vi "Drive Controller.vi"(8 "error in":errorcluster) -> ()   [LabVIEW 2020]
doc: "This VI executes continuously carrying out the current operation and responding to updates or new operation requests. It will often contain the timing or control code that is difficult to place directly in TeleOp. This VI generally opens all sensors and motors and isolates the rest of the robot code from knowing implementation details of how the operations are carried out."
uses:
  <vilib>/Rock Robotics/WPI/Framework/Completion Status.ctl
  Drive Setpoints.ctl
  Drive Operations.ctl
  <vilib>/Rock Robotics/WPI/SafetyOutput/WPI_SafetyOutputConfigMenu.ctl
  <vilib>/Rock Robotics/WPI/Utilities/WPI_GetSetVariantRefNum.vi
  <vilib>/Rock Robotics/Network Tables/NT Write Number.vi
panel:
  in  "Interactive Values":T1
  in  "Buttons":cluster{"Execute Cmd":bool, "Abort Cmd":bool}
  out "Command Timing":cluster{"Start Time (ms)":u32, "Iterations":i32}
  out "Status":T3
  out "Setpoints":T4(graph)
  out "Current\nCmd":string
  # "Tip: The graph shows the motor setpoints. It may also be helpful to observe inputs and sensor values.\nYou may also want to display tuning or debugging controls."
  # "Interactive Command: You may fill in the settings for a command\nand schedule it with the Execute button. You can observe and abort\nany command while fine tuning the code for the controller."
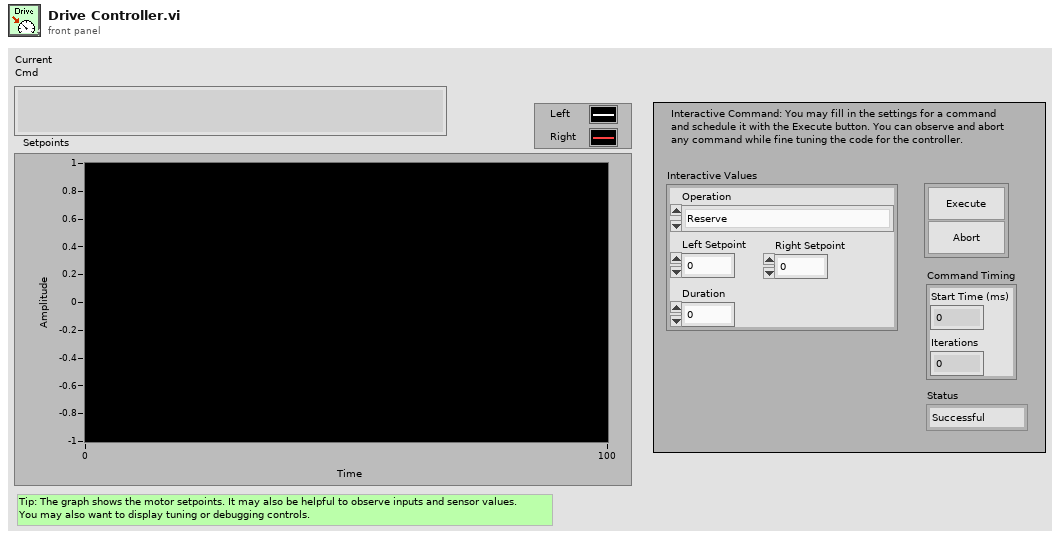
[diagram p1: front panel]
types:
  T1 = typedef "Drive Setpoints.ctl" = cluster{"Operation":T2, "Left Setpoint":dbl, "Right Setpoint":dbl, "Duration":dbl}
  T2 = typedef "Drive Operations.ctl" = enum16{"Reserve", "Read Current", "Immediate", "Drive for Time", "Drive for Distance"}
  T3 = typedef "Completion Status.ctl" = enum16{"Successful", "Aborted", "Incomplete"}
  T4 = cluster{"Left Setpoint":dbl, "Right Setpoint":dbl}
  T5 = typedef "WPI_SafetyOutputConfigMenu.ctl" = enum16{"Enable", "Disable"}
  T6 = typedef "WPI_RobotDriveDevRef.ctl" = cluster{"DevStatus":errorcluster, "Motors[]":T7[], "Square Inputs":bool, "Max Output":dbl}
  T7 = typedef "WPI_MotorControlDeviceRef.ctl" = cluster{"DeviceStatus":errorcluster, "Type":T8, "PWM":cluster{"PWM Channel":T9, "DeadBand":T10}, "CAN":cluster{"Device Number":u8, "SetOutput VI Ref":variant, "GetOutput VI Ref":variant, "Enable VI Ref":variant, "Disable VI Ref":variant, "Data":variant}, "Invert":bool, "DIO PWM":cluster{"PWM \"Enable\" Channel":T9, "DIOChannel":T11, "PWM Rate":dbl}}
  T8 = typedef "WPI_MotorControlType.ctl" = enum16{"PWM", "CAN", "DIO PWM"}
  T9 = typedef "FPGA_DIOPWMChannel.ctl" = enum8{"PWM 0", "PWM 1", "PWM 2", "PWM 3", "PWM 4", "PWM 5", "PWM 6", "PWM 7", "PWM 8", "PWM 9", "PWM MXP 0", "PWM MXP 1", "PWM MXP 2", "PWM MXP 3", "PWM MXP 4", "PWM MXP 5", "PWM MXP 6", "PWM MXP 7", "PWM MXP 8", "PWM MXP 9", "Invalid"}
  T10 = typedef "WPI_PWMDeadband.ctl" = cluster{"Name":string, "maxPositivePwm":i32, "minPositivePwm":i32, "centerPwm":i32, "maxNegativePwm":i32, "minNegativePwm":i32, "angularRange":u16}
  T11 = typedef "FPGA_DIOChannel.ctl" = enum8{"DIO 0", "DIO 1", "DIO 2", "DIO 3", "DIO 4", "DIO 5", "DIO 6", "DIO 7", "DIO 8", "DIO 9", "DIO MXP 0", "DIO MXP 1", "DIO MXP 2", "DIO MXP 3", "DIO MXP 4", "DIO MXP 5", "DIO MXP 6", "DIO MXP 7", "DIO MXP 8", "DIO MXP 9", "DIO MXP 10", "DIO MXP 11", "DIO MXP 12", "DIO MXP 13", "DIO MXP 14", "DIO MXP 15", "SPI Port CS1", "SPI Port CS2", "SPI Port CS3", "SPI Port MISO", "SPI Port MOSI", "Invalid"}
  T12 = typedef "Command Status Info.ctl" = cluster{"Name":string, "Status":T3, "notifier out":T13}
  T13 = typedef "Completion Notifier.ctl" = refnum<notifier>
  T14 = cluster{"SubSystem Data":T1, cluster{"Start Time (ms)":u32, "Iterations":i32}, cluster{"Command Info":T12, "Description":string, "Default Command":T1, "queue out":refnum<queue>, "Subsystem Name":string}}
  T15 = cluster{"SubSystem Data":T1, cluster{"Start Time (ms)":u32, "Iterations":i32}, "Default Command Arguments":cluster{"Command Info":T12, "Description":string, "Default Command":T1, "queue out":refnum<queue>, "Subsystem Name":string}}
  T16 = cluster{"Don't move motors while reserved":dbl, "Don't move motors while reserved":dbl}
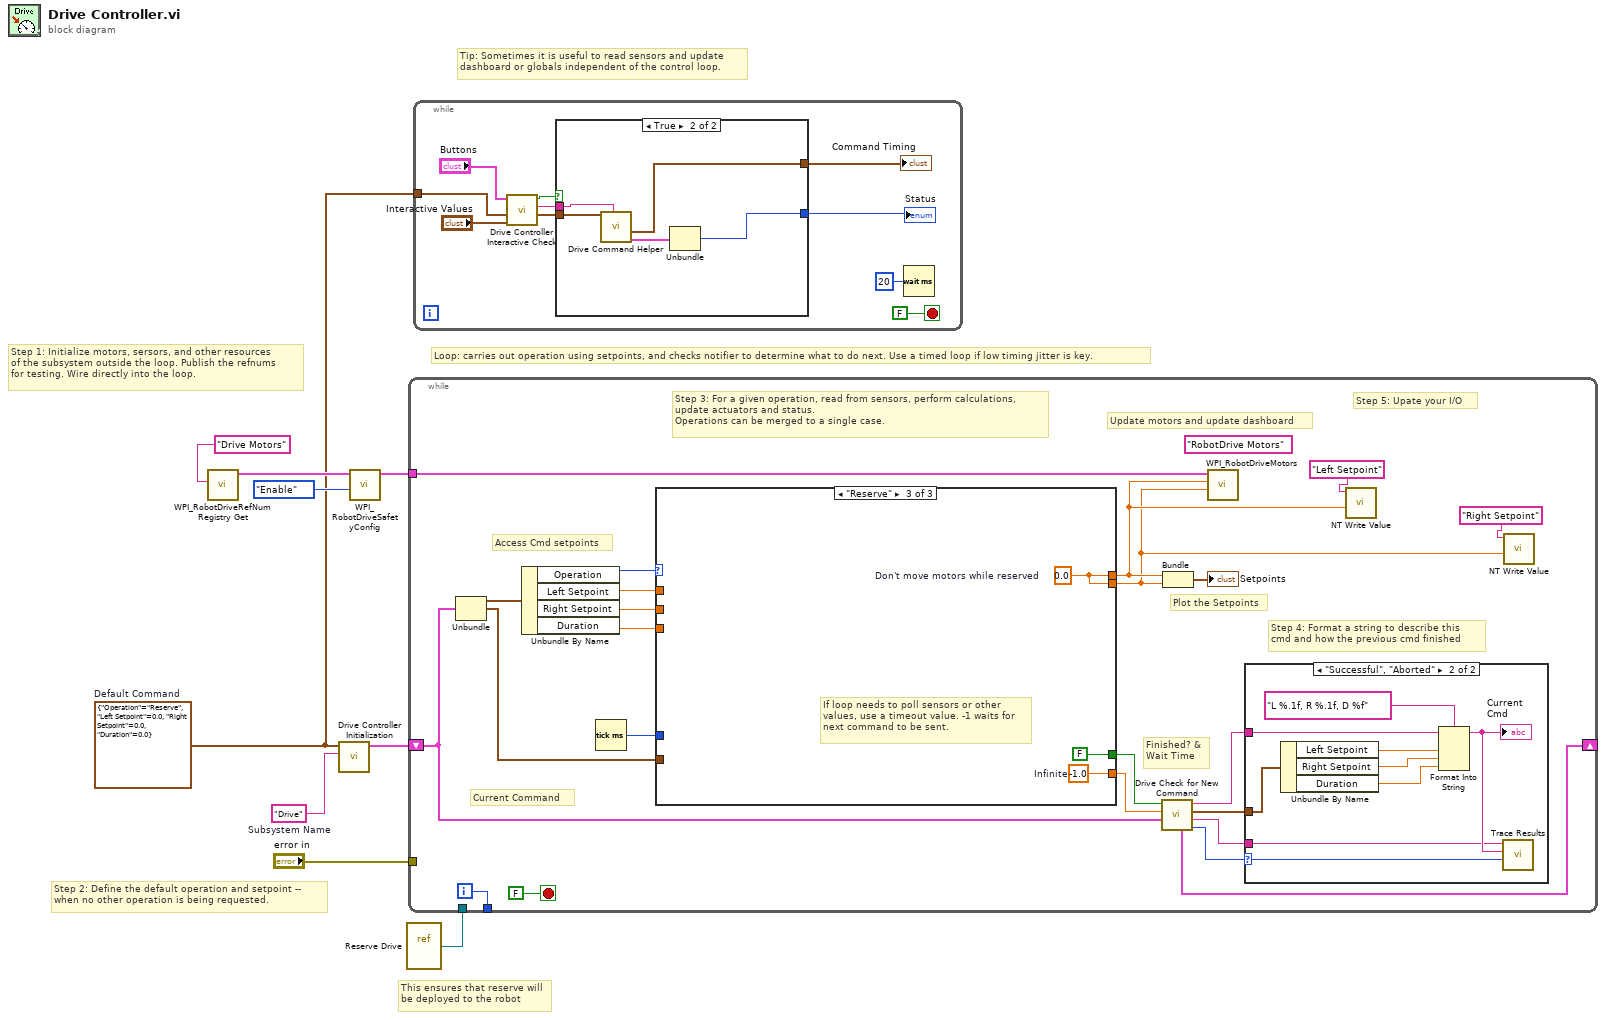
[diagram p0: block diagram]
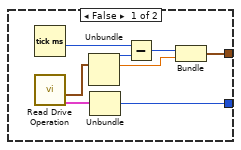
[diagram p2: hidden frame]
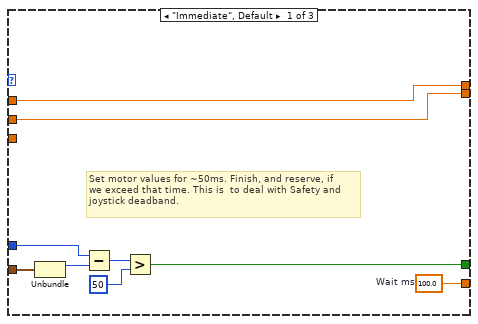
[diagram p4: hidden frame]
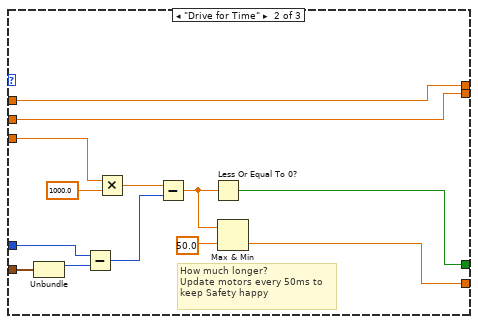
[diagram p5: hidden frame]
diagram:
  w1 = T1 {"Operation"=enum."Reserve", "Left Setpoint"=0.0, "Right Setpoint"=0.0, "Duration"=0.0}  # Default Command
  w9 = "Drive"  # Subsystem Name
  # "This ensures that reserve will\nbe deployed to the robot"
  # "Tip: Sometimes it is useful to read sensors and update\ndashboard or globals independent of the control loop."
  # "Step 2: Define the default operation and setpoint --\nwhen no other operation is being requested."
  # "Step 1: Initialize motors, sersors, and other resources\nof the subsystem outside the loop. Publish the refnums\nfor testing. Wire directly into the loop."
  # "Loop: carries out operation using setpoints, and checks notifier to determine what to do next. Use a timed loop if low timing jitter is key."
  n1 = call <vilib>:"WPI_RobotDriveRefNum Registry Get.vi"("refnum name"="Drive Motors") -> ("RobotDriveDevRef"=w7:T6)  [unwired: 9 in, 1 out]
  n2 = call "Drive Controller Initialization.vi"("Subsystem Name"=w9, "Default Command"=w1) -> ("Current Command"=w3:T14)  [unwired: 9 in]
  n3 = call <vilib>:"WPI_RobotDriveSafetyConfig.vi"("mode"=WPI_SafetyOutputConfigMenu."Enable", "RobotDriveDevRef"=w7) -> ("RobotDriveDevRef"=w5:T6)  [unwired: 8 in, 1 out]
  n4 = vi-ref "Reserve Drive.vi"() -> (w2:refnum<vi>)
  n5 = while {
    shift-right: [w21] -> _
    shift-left: w3 -> [w14]
    tunnel: [w31] -> _
    tunnel: w5 -> [w29]
    tunnel: "error in" -> [_]
    tunnel: w2 -> [_]
    i -> [w31]
    stop <- FALSE stop-if-true
    (unwired) "RobotDrive Motors" ("Name")
    # "Step 5: Upate your I/O"
    # "Step 4: Format a string to describe this\ncmd and how the previous cmd finished"
    # "Current Command"
    # "Update motors and update dashboard"
    # "Plot the Setpoints"
    # "Access Cmd setpoints"
    # "Finished? &\nWait Time"
    # "Step 3: For a given operation, read from sensors, perform calculations,\nupdate actuators and status.\nOperations can be merged to a single case."
    n6 = Unbundle(w14) -> ("SubSystem Data"=w28:T1, w15:cluster{"Start Time (ms)":u32, "Iterations":i32})  [unwired: 1 out]
    n7 = Unbundle By Name(w28) -> ("Operation"=w27:T2, "Left Setpoint"=w26:dbl, "Right Setpoint"=w25:dbl, "Duration"=w24:dbl)
    n8 = Tick Count (ms)() -> (millisecond timer value=w23:u32)
    n9 = case shown="\"Reserve\"" w27 {
      tunnel: [w50 w51 w66] -> w20
      tunnel: [w43 w58 FALSE ("ignore previous (F)")] -> w19
      tunnel: w15 -> [w42 w60 _]
      tunnel: [w49 w57 w64] -> w11
      tunnel: [w48 w56 w64] -> w10
      tunnel: w26 -> [w49 w57 _]
      tunnel: w25 -> [w48 w56 _]
      tunnel: w24 -> [_ w55 _]
      tunnel: w23 -> [w44 w54 _]
      frame "Immediate", Default {
        w50 = 100.0  # Wait ms
        # "Set motor values for ~50ms. Finish, and reserve, if\nwe exceed that time. This is  to deal with Safety and\njoystick deadband."
        n10 = Unbundle(w42) -> ("Start Time (ms)"=w45:u32)  [unwired: 1 out]
        n11 = Subtract(x=w44, y=w45) -> (x-y=w46:u32)
        n12 = Greater?(x=w46, y=u8 50 ("Left Motor")) -> (0:w43:bool)
      }
      frame "Drive for Time" {
        # "How much longer?\nUpdate motors every 50ms to\nkeep Safety happy"
        n13 = Unbundle(w60) -> ("Start Time (ms)"=w59:u32)  [unwired: 1 out]
        n14 = Subtract(x=w54, y=w59) -> (x-y=w63:u32)
        n15 = Multiply(x=w55, y=1000.0) -> (x*y=w62:dbl)
        n16 = Subtract(x=w62, y=w63) -> (x-y=w53:dbl)
        n17 = Less Or Equal To 0?(x=w53) -> (x <= 0?=w58:bool)
        n18 = Max & Min(x=w53, y=50.0) -> (min(x,y)=w51:dbl)  [unwired: 1 out]
      }
      frame "Reserve" {
        w64 = 0.0  # Don't move motors while reserved
        w66 = -1.0  # Infinite
        # "If loop needs to poll sensors or other\nvalues, use a timeout value. -1 waits for\nnext command to be sent."
      }
    }
    n19 = call "Drive Check for New Command.vi"("input cluster"=w14, "Wait time (ms)"=w20, "Finished?"=w19) -> ("Completion"=w22:T3, "Subsystem Name"=w16:string, "Current Command"=w17:T1, "Initial Trace String"=w18:string, "Next Command"=w21:T15)  [unwired: 4 in]
    n20 = Bundle("Don't move motors while reserved"=w11, "Don't move motors while reserved"=w10) -> (→"Setpoints":T16)  [unwired: 1 in]
    n21 = call <vilib>:"WPI_RobotDriveMotors.vi"("RightSpeed"=w10, "LeftSpeed"=w11, "RobotDriveDevRef"=w29) -> ()  [unwired: 1 in, 8 out]
    n22 = case shown="\"Successful\", \"Aborted\"" w22 {
      selector: w22 -> [_ w41]
      tunnel: w18 -> [_ w36]
      tunnel: w17 -> [_ w37]
      tunnel: w16 -> [_ w33]
      frame "Incomplete", Default {
        # "Continuing current command"
      }
      frame "Successful", "Aborted" {
        # "Report and setup for next command"
        n23 = Unbundle By Name(w37) -> ("Left Setpoint"=w39:dbl, "Right Setpoint"=w40:dbl, "Duration"=w34:dbl)
        n24 = Format Into String(format string="L %.1f, R %.1f, D %f", initial string=w36, w39, w40, w34) -> (resulting string=w35:string)  [unwired: 1 in, 1 out]
        "Current\nCmd" <- w35
        n25 = call <vilib>:"Trace Results.vi"("Status of previous command"=w41, "Description"=w35, "Subsystem"=w33) -> ()  [unwired: 9 in]
      }
    }
    n26 = call-poly <vilib>:"NT Write Value.vi"("Numeric"=w11, "Name"="Left Setpoint") -> ()  [unwired: 9 in, 1 out]
    n27 = call-poly <vilib>:"NT Write Value.vi"("Numeric"=w10, "Name"="Right Setpoint") -> ()  [unwired: 9 in, 1 out]
  }
  n28 = while {
    tunnel: w1 -> [w68]
    stop <- FALSE stop-if-true
    n29 = call "Drive Controller Interactive Check.vi"("Interactive Command In"="Interactive Values", "Default Command"=w68, "Buttons"="Buttons") -> ("Interactive Command Out"=w70:T1, "Trace String"=w71:string, "Schedule"=w72:bool)  [unwired: 6 in]
    n30 = case shown="True" w72 {
      tunnel: [w81 w89] -> w73
      tunnel: [w80 w85] -> w74
      tunnel: w71 -> [_ w87]
      tunnel: w70 -> [_ w86]
      frame False {
        n31 = Tick Count (ms)() -> (millisecond timer value=w84:u32)
        n32 = call "Read Drive Operation.vi"() -> ("Command Info"=w78:T12, "SubSystem Data"=w77:T1)  [unwired: 9 in, 1 out]
        n33 = Unbundle(w77) -> ("Operation"=w82:T2, "Left Setpoint"=w79:dbl)  [unwired: 2 out]
        n34 = Unbundle(w78) -> ("Status"=w81:T3)  [unwired: 2 out]
        n35 = Subtract(x=w84, y=w82) -> (x-y=w83:u32)
        n36 = Bundle(w83, "Left Setpoint"=w79) -> (w80:cluster{u32, "Left Setpoint":dbl})  [unwired: 1 in]
      }
      frame True {
        n37 = call "Drive Command Helper.vi"("Description"=w87, "SubSystem Data"=w86) -> ("Command Info Out"=w88:T12, "Command Timing"=w85:cluster{"Start Time (ms)":u32, "Iterations":i32})  [unwired: 7 in, 1 out]
        n38 = Unbundle(w88) -> ("Status"=w89:T3)  [unwired: 2 out]
      }
    }
    "Status" <- w73
    "Command Timing" <- w74
    n39 = Wait (ms)(milliseconds to wait=u32 20) -> ()  [unwired: 1 out]
  }
